vi "V3-adam-write-&-check-response.vi"(8 "error in (no error)":errorcluster, 10 "write buffer":string, 11 "VISA resource name":refnum<visa-resource-name>) -> (0 "error out":errorcluster, 1 "cmd aknowledged":bool, 2 "acknowledge char":string, 3 "VISA resource name out":refnum<visa-resource-name>, 4 "read buffer":string)   [LabVIEW 2020]
panel:
  out "String":string="\r"
  out "(cr)":bool
  out "string-builder":string
  out "last-char":string
  out "return count":u32
  out "number pause loops":i32
  out "No. Bytes at Port":u32
  out "read return":u32
  out "pause-time":u32
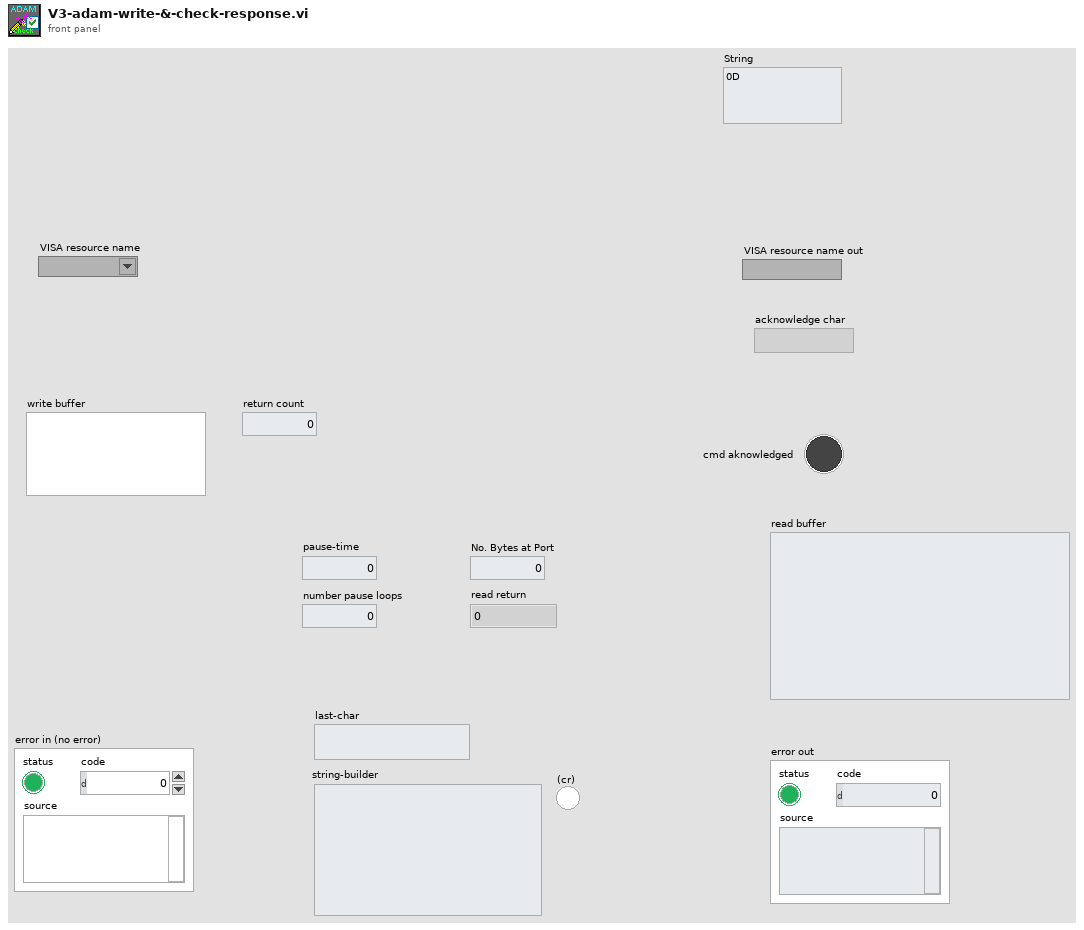
[diagram p1: front panel]
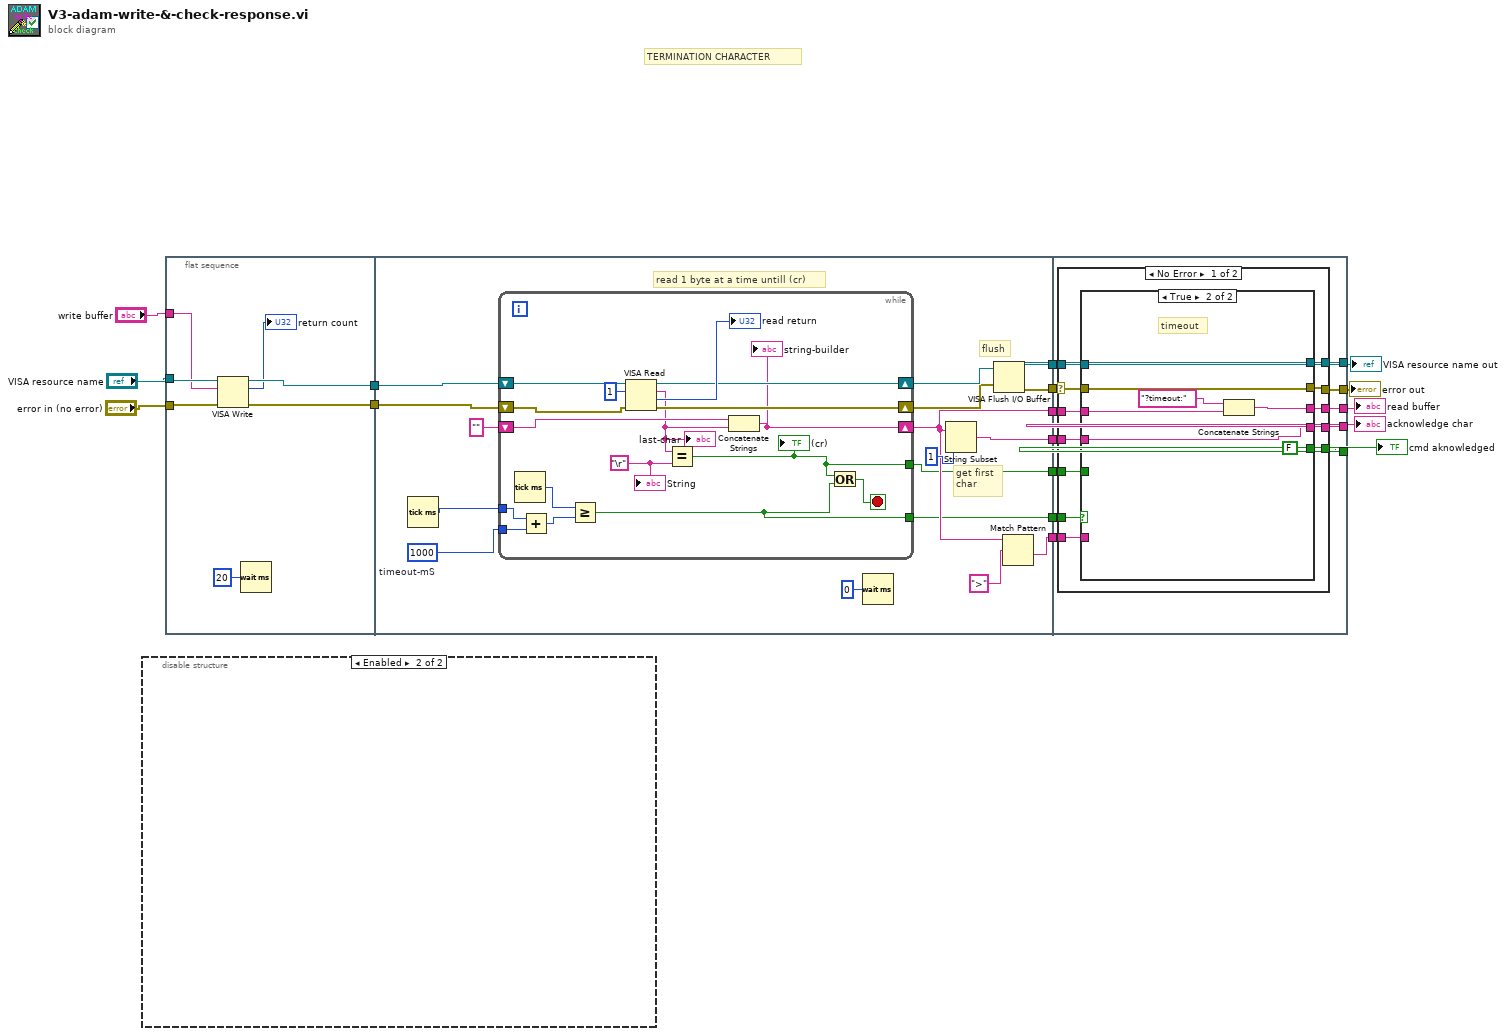
[diagram p0: block diagram]
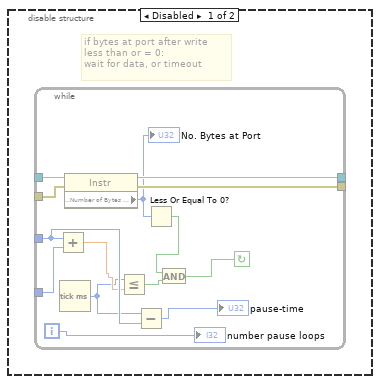
[diagram p2: hidden frame]
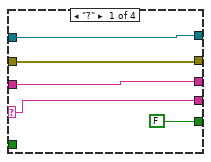
[diagram p4: hidden frame]
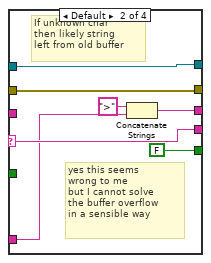
[diagram p5: hidden frame]
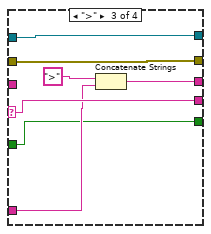
[diagram p6: hidden frame]
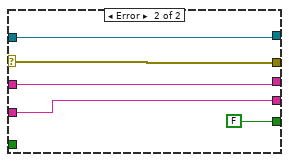
[diagram p7: hidden frame]
diagram:
  # "TERMINATION CHARACTER"
  n1 = disable-structure shown="Enabled" {
    frame Disabled {
      # "if bytes at port after write\nless than or = 0:\nwait for data, or timeout"
      n2 = while {
        tunnel: [w31] -> _
        tunnel: [w30] -> _
        tunnel: _ -> [w25]
        tunnel: _ -> [w29]
        tunnel: _ -> [w24]
        tunnel: _ -> [w23]
        i -> [w19]
        stop <- w28 continue-if-true
        n3 = Add(x=w25, y=w29) -> (x+y=w22:dbl)
        n4 = Tick Count (ms)() -> (millisecond timer value=w21:u32)
        n5 = property class="Instr"(reference=w23, error in=w24) -> (reference out=w31:refnum<visa-resource-name>, error out=w30:errorcluster, "Serial Settings:Number of Bytes at Serial Port"=w20:u32)
        "No. Bytes at Port" <- w20
        n6 = Less Or Equal?(x=w21, y=w22) -> (x <= y?=w26:bool)
        n7 = Subtract(x=w21, y=w25) -> (x-y=→"pause-time":u32)
        n8 = Less Or Equal To 0?(x=w20) -> (x <= 0?=w27:bool)
        n9 = And(x=w27, y=w26) -> (x .and. y?=w28:bool)
        "number pause loops" <- w19
      }
    }
    frame Enabled {
    }
  }
  n10 = flat-sequence {
    tunnel: "error in (no error)" -> [w37]
    tunnel: "VISA resource name" -> [w38]
    tunnel: "write buffer" -> [w32]
    tunnel: [w36] -> w7
    tunnel: [w35] -> w6
    tunnel: [w48] -> w14
    tunnel: [w54] -> w13
    tunnel: [w53] -> w12
    tunnel: w7 -> [w43]
    tunnel: w6 -> [w44]
    tunnel: [w47] -> w5
    tunnel: [w46] -> w3
    tunnel: [w40] -> w2
    tunnel: [w39] -> w1
    tunnel: w14 -> [w83]
    tunnel: w13 -> [w84]
    tunnel: w12 -> [w82]
    tunnel: [w81] -> w11
    tunnel: [w80] -> w10
    tunnel: [w79] -> w9
    tunnel: [w78] -> w8
    tunnel: w5 -> [w77]
    tunnel: [w76] -> w4
    tunnel: w3 -> [w75]
    tunnel: w2 -> [w74]
    tunnel: w1 -> [w73]
    frame #0 {
      n11 = VISA Write(VISA resource name=w38, write buffer=w32, error in (no error)=w37) -> (VISA resource name out=w35:refnum<visa-resource-name>, return count=→"return count":u32, error out=w36:errorcluster)
      n12 = Wait (ms)(milliseconds to wait=u32 20) -> ()  [unwired: 1 out]
    }
    frame #1 {
      w41 = u32 1000  # timeout-mS
      # "read 1 byte at a time untill (cr)"
      # "get first\nchar"
      # "flush"
      n13 = Tick Count (ms)() -> (millisecond timer value=w42:u32)
      n14 = while {
        shift-right: [w71] -> w52
        shift-left: w44 -> [w66]
        shift-right: [w70] -> w51
        shift-left: w43 -> [w67]
        shift-right: [w68] -> w46
        shift-left: "" ("read buffer") -> [w69]
        tunnel: w42 -> [w60]
        tunnel: w41 -> [w61]
        tunnel: [w57] -> w40
        tunnel: [w56] -> w39
        stop <- w62 stop-if-true
        w63 = "\r"
        n15 = Tick Count (ms)() -> (millisecond timer value=w59:u32)
        n16 = Add(x=w60, y=w61) -> (x+y=w58:u32)
        n17 = Greater Or Equal?(x=w59, y=w58) -> (x >= y?=w56:bool)
        n18 = VISA Read(VISA resource name=w66, byte count=u32 1, error in (no error)=w67) -> (VISA resource name out=w71:refnum<visa-resource-name>, read buffer=w64:string, return count=→"read return":u32, error out=w70:errorcluster)
        "last-char" <- w64
        n19 = Equal?(x=w64, y=w63) -> (x = y?=w57:bool)
        "(cr)" <- w57
        n20 = Concatenate Strings(w69, w64) -> (w68:string)
        "string-builder" <- w68
        n21 = Or(x=w57, y=w56) -> (x .or. y?=w62:bool)
        "String" <- w63
      }
      n22 = Wait (ms)(milliseconds to wait=u32 0) -> ()  [unwired: 1 out]
      n23 = String Subset(string=w46, length (rest)=1 ("length (rest)")) -> (substring=w48:string)  [unwired: 1 in]
      n24 = VISA Flush I/O Buffer(VISA resource name=w52, error in (no error)=w51) -> (VISA resource name out=w53:refnum<visa-resource-name>, error out=w54:errorcluster)  [unwired: 1 in]
      n25 = Match Pattern(string=w46, regular expression=">") -> (after substring=w47:string)  [unwired: 1 in, 3 out]
    }
    frame #2 {
      n26 = case shown="No Error" w84 {
        selector: w84 -> [w92 w143]
        tunnel: [w96 FALSE ("cmd aknowledged")] -> w81
        tunnel: w83 -> [w95 w142]
        tunnel: [w94 w142] -> w80
        tunnel: [w93 w143] -> w79
        tunnel: w82 -> [w91 w140]
        tunnel: [w90 w140] -> w78
        tunnel: w77 -> [w89 _]
        tunnel: [w88 w139] -> w76
        tunnel: w75 -> [w87 w139]
        tunnel: w74 -> [w86 _]
        tunnel: w73 -> [w85 _]
        frame No Error {
          n27 = case shown="True" w85 {
            tunnel: [w107 FALSE ("cmd aknowledged")] -> w96
            tunnel: w95 -> [w106 w132]
            tunnel: [w105 w132] -> w94
            tunnel: [w104 w137] -> w93
            tunnel: w92 -> [w103 w137]
            tunnel: w91 -> [w102 w136]
            tunnel: [w101 w136] -> w90
            tunnel: w89 -> [w100 _]
            tunnel: [w99 w133] -> w88
            tunnel: w87 -> [w98 w135]
            tunnel: w86 -> [w97 _]
            frame False {
              n28 = case shown="\"!\"" w106 {
                selector: w106 -> [w111 w118 w126 w131]
                tunnel: [FALSE ("cmd aknowledged") FALSE ("cmd aknowledged") w120 w127] -> w107
                tunnel: [w111 w118 w126 w131] -> w105
                tunnel: [w110 w117 w125 w130] -> w104
                tunnel: w103 -> [w110 w117 w125 w130]
                tunnel: w102 -> [w109 w116 w124 w129]
                tunnel: [w109 w116 w124 w129] -> w101
                tunnel: w100 -> [_ w114 w123 _]
                tunnel: [w108 w115 w122 w128] -> w99
                tunnel: w98 -> [w108 _ _ w128]
                tunnel: w97 -> [_ _ w120 w127]
                frame "?" {
                }
                frame Default {
                  # "yes this seems\nwrong to me\nbut I cannot solve \nthe buffer overflow \nin a sensible way"
                  # "If unknown char\nthen likely string\nleft from old buffer"
                  n29 = Concatenate Strings(">" ("string"), w114) -> (w115:string)
                }
                frame ">" {
                  n30 = Concatenate Strings(">" ("string"), w123) -> (w122:string)
                }
                frame "!" {
                }
              }
            }
            frame True {
              # "timeout"
              n31 = Concatenate Strings("?timeout:", w135) -> (w133:string)
            }
          }
        }
        frame Error {
        }
      }
    }
  }
  "error out" <- w9
  "VISA resource name out" <- w8
  "cmd aknowledged" <- w11
  "acknowledge char" <- w10
  "read buffer" <- w4
